vi "Lab Panel V5.24.1.vi"() -> ()   [LabVIEW 2013] (continued)
                n1784 = property on="O/I  LAB02-2" class="Bool (strict)"("DisabledEnum"=w3327) -> ()  [unwired: 2 in, 2 out]
                n1785 = property on="O/I  LAB03-1" class="Bool (strict)"("DisabledEnum"=w3326) -> ()  [unwired: 2 in, 2 out]
              }
              frame #1 {
                n1786 = Select(t=2, s=w3360, f=0) -> (s? t:f=w3351:i32)
                n1787 = Select(t=2, s=w3359, f=0) -> (s? t:f=w3352:i32)
                n1788 = Select(t=2, s=w3356, f=0) -> (s? t:f=w3355:i32)
                n1789 = Select(t=2, s=w3357, f=0) -> (s? t:f=w3354:i32)
                n1790 = Select(t=2, s=w3358, f=0) -> (s? t:f=w3353:i32)
                n1791 = property on="SELECT LAB05-2" class="RadioBtnsControl (strict)"("DisabledEnum"=w3351) -> ()  [unwired: 2 in, 2 out]
                n1792 = property on="SELECT LAB05-1" class="RadioBtnsControl (strict)"("DisabledEnum"=w3352) -> ()  [unwired: 2 in, 2 out]
                n1793 = property on="SELECT LAB03-2" class="RadioBtnsControl (strict)"("DisabledEnum"=w3355) -> ()  [unwired: 2 in, 2 out]
                n1794 = property on="SELECT LAB04-1" class="RadioBtnsControl (strict)"("DisabledEnum"=w3354) -> ()  [unwired: 2 in, 2 out]
                n1795 = property on="SELECT LAB04-2" class="RadioBtnsControl (strict)"("DisabledEnum"=w3353) -> ()  [unwired: 2 in, 2 out]
                n1796 = property on="SET LAB05-2" class="Clust (strict)"("DisabledEnum"=w3351) -> ()  [unwired: 2 in, 2 out]
                n1797 = property on="SET LAB05-1" class="Clust (strict)"("DisabledEnum"=w3352) -> ()  [unwired: 2 in, 2 out]
                n1798 = property on="SET LAB03-2" class="Clust (strict)"("DisabledEnum"=w3355) -> ()  [unwired: 2 in, 2 out]
                n1799 = property on="SET LAB04-1" class="Clust (strict)"("DisabledEnum"=w3354) -> ()  [unwired: 2 in, 2 out]
                n1800 = property on="SET LAB04-2" class="Clust (strict)"("DisabledEnum"=w3353) -> ()  [unwired: 2 in, 2 out]
                n1801 = property on="O/I  LAB05-2" class="Bool (strict)"("DisabledEnum"=w3351) -> ()  [unwired: 2 in, 2 out]
                n1802 = property on="O/I  LAB05-1" class="Bool (strict)"("DisabledEnum"=w3352) -> ()  [unwired: 2 in, 2 out]
                n1803 = property on="O/I  LAB04-1" class="Bool (strict)"("DisabledEnum"=w3354) -> ()  [unwired: 2 in, 2 out]
                n1804 = property on="O/I  LAB04-2" class="Bool (strict)"("DisabledEnum"=w3353) -> ()  [unwired: 2 in, 2 out]
                n1805 = property on="O/I  LAB03-2" class="Bool (strict)"("DisabledEnum"=w3355) -> ()  [unwired: 2 in, 2 out]
                n1806 = Not(x=w3360) -> (.not. x?=w3361:bool)
                n1807 = Not(x=w3359) -> (.not. x?=w3362:bool)
                n1808 = Not(x=w3358) -> (.not. x?=w3363:bool)
                n1809 = property on="RESULT LAB05-2" class="Bool (strict)"("Visible"=w3361) -> ()  [unwired: 2 in, 2 out]
                n1810 = property on="RESULT LAB05-1" class="Bool (strict)"("Visible"=w3362) -> ()  [unwired: 2 in, 2 out]
                n1811 = Not(x=w3357) -> (.not. x?=w3364:bool)
                n1812 = property on="RESULT LAB04-2" class="Bool (strict)"("Visible"=w3363) -> ()  [unwired: 2 in, 2 out]
                n1813 = Not(x=w3356) -> (.not. x?=w3365:bool)
                n1814 = property on="RESULT LAB04-1" class="Bool (strict)"("Visible"=w3364) -> ()  [unwired: 2 in, 2 out]
                n1815 = property on="RESULT LAB03-2" class="Bool (strict)"("Visible"=w3365) -> ()  [unwired: 2 in, 2 out]
              }
              frame #2 {
                # "disable calibrate if any test running"
                n1816 = Or(x=w3388, y=w3387) -> (x .or. y?=w3381:bool)
                n1817 = Or(x=w3390, y=w3389) -> (x .or. y?=w3383:bool)
                n1818 = Or(x=w3394, y=w3393) -> (x .or. y?=w3385:bool)
                n1819 = Or(x=w3392, y=w3391) -> (x .or. y?=w3384:bool)
                n1820 = Or(x=w3396, y=w3395) -> (x .or. y?=w3386:bool)
                n1821 = Or(x=w3384, y=w3383) -> (x .or. y?=w3382:bool)
                n1822 = Or(x=w3386, y=w3385) -> (x .or. y?=w3380:bool)
                n1823 = Or(x=w3382, y=w3381) -> (x .or. y?=w3379:bool)
                n1824 = Or(x=w3380, y=w3379) -> (x .or. y?=w3376:bool)
                "Any Test Running" <- w3376
                n1825 = case shown="False" w3376 {
                  tunnel: [0 2] -> w3378
                  frame False {
                  }
                  frame True {
                  }
                }
                n1826 = property on="JIG TEST" class="Clust (strict)"("DisabledEnum"=w3378) -> ()  [unwired: 2 in, 2 out]
                n1827 = property on="Network Directory" class="Path"("DisabledEnum"=w3378) -> ()  [unwired: 2 in, 2 out]
                n1828 = property on="MAIL SETTINGS" class="Clust (strict)"("DisabledEnum"=w3378) -> ()  [unwired: 2 in, 2 out]
                n1829 = property on="SET (cal)" class="Bool (strict)"("DisabledEnum"=w3378) -> ()  [unwired: 2 in, 2 out]
                n1830 = property on="ADMIN" class="Bool (strict)"("DisabledEnum"=0) -> ()  [unwired: 2 in, 2 out]
              }
            }
          }
          frame #8 {
            # "drive jigs"
            n1831 = stacked-sequence {
              frame #0 {
                # "jig on"
                n1832 = local read "jig cycle"() -> (w3404:dbl)
                n1833 = property on="JIG TEST" class="Clust (strict)"() -> ("DisabledEnum"=w3401:T16)  [unwired: 2 in, 2 out]
                n1834 = Equal?(x=w3401, y=2) -> (x = y?=w3400:bool)
                n1835 = Equal?(x=w3404, y=0) -> (x = y?=w3402:bool)
                n1836 = And(x=w3402, y=w3400) -> (x .and. y?=w3399:bool)
                n1837 = case shown="True" w3399 {
                  frame False {
                  }
                  frame True {
                    n1838 = local read "run lab01-1"() -> (w3415:bool)
                    n1839 = local read "run lab01-2"() -> (w3414:bool)
                    n1840 = local read "run lab02-1"() -> (w3413:bool)
                    n1841 = local read "run lab02-2"() -> (w3412:bool)
                    n1842 = local read "run lab03-1"() -> (w3411:bool)
                    n1843 = local read "run lab03-2"() -> (w3410:bool)
                    n1844 = local read "run lab04-1"() -> (w3409:bool)
                    n1845 = local read "run lab04-2"() -> (w3408:bool)
                    n1846 = local read "run lab05-1"() -> (w3407:bool)
                    n1847 = local read "run lab05-2"() -> (w3406:bool)
                    n1848 = local write "JIG LAB03-2"(w3410) -> ()
                    n1849 = local write "JIG LAB01-1"(w3415) -> ()
                    n1850 = local write "JIG LAB01-2"(w3414) -> ()
                    n1851 = local write "JIG LAB02-1"(w3413) -> ()
                    n1852 = local write "JIG LAB02-2"(w3412) -> ()
                    n1853 = local write "JIG LAB03-1"(w3411) -> ()
                    n1854 = local write "JIG LAB04-1"(w3409) -> ()
                    n1855 = local write "JIG LAB04-2"(w3408) -> ()
                    n1856 = local write "JIG LAB05-1"(w3407) -> ()
                    n1857 = local write "JIG LAB05-2"(w3406) -> ()
                  }
                }
              }
              frame #1 {
                # "jig off"
                n1858 = local read "jig cycle"() -> (w3422:dbl)
                n1859 = local read "on loops"() -> (w3421:dbl)
                n1860 = property on="JIG TEST" class="Clust (strict)"() -> ("DisabledEnum"=w3420:T16)  [unwired: 2 in, 2 out]
                n1861 = Equal?(x=w3420, y=2) -> (x = y?=w3418:bool)
                n1862 = Equal?(x=w3422, y=w3421) -> (x = y?=w3417:bool)
                n1863 = And(x=w3417, y=w3418) -> (x .and. y?=w3416:bool)
                n1864 = case shown="True" w3416 {
                  frame False {
                  }
                  frame True {
                    w3473 = FALSE
                    w3474 = TRUE
                    w3472 = 2
                    n1865 = local read "SELECT LAB05-2"() -> (w3463:T3)
                    n1866 = local read "SELECT LAB04-2"() -> (w3465:T3)
                    n1867 = local read "SELECT LAB04-1"() -> (w3466:T3)
                    n1868 = local read "SELECT LAB05-1"() -> (w3464:T3)
                    n1869 = local read "SELECT LAB03-2"() -> (w3467:T3)
                    n1870 = local read "SELECT LAB02-1"() -> (w3470:T3)
                    n1871 = local read "SELECT LAB03-1"() -> (w3468:T3)
                    n1872 = local read "SELECT LAB02-2"() -> (w3469:T3)
                    n1873 = local read "SELECT LAB01-2"() -> (w3471:T3)
                    n1874 = local read "run lab05-1"() -> (w3433:bool)
                    n1875 = local read "run lab05-2"() -> (w3432:bool)
                    n1876 = local read "SELECT LAB01-1"() -> (w3475:T3)
                    n1877 = local read "run lab04-2"() -> (w3434:bool)
                    n1878 = local read "run lab04-1"() -> (w3435:bool)
                    n1879 = local read "run lab01-1"() -> (w3451:bool)
                    n1880 = local read "run lab01-2"() -> (w3440:bool)
                    n1881 = local read "run lab03-2"() -> (w3436:bool)
                    n1882 = local read "run lab03-1"() -> (w3437:bool)
                    n1883 = local read "run lab02-1"() -> (w3439:bool)
                    n1884 = local read "run lab02-2"() -> (w3438:bool)
                    n1885 = Equal?(x=w3472, y=w3468) -> (x = y?=w3446:bool)
                    n1886 = Equal?(x=w3472, y=w3467) -> (x = y?=w3445:bool)
                    n1887 = Equal?(x=w3472, y=w3466) -> (x = y?=w3444:bool)
                    n1888 = Equal?(x=w3472, y=w3465) -> (x = y?=w3443:bool)
                    n1889 = Equal?(x=w3472, y=w3464) -> (x = y?=w3442:bool)
                    n1890 = Equal?(x=w3472, y=w3463) -> (x = y?=w3441:bool)
                    n1891 = Equal?(x=w3472, y=w3475) -> (x = y?=w3452:bool)
                    n1892 = Equal?(x=w3472, y=w3470) -> (x = y?=w3448:bool)
                    n1893 = Equal?(x=w3472, y=w3469) -> (x = y?=w3447:bool)
                    n1894 = Equal?(x=w3472, y=w3471) -> (x = y?=w3449:bool)
                    n1895 = And(x=w3443, y=w3434) -> (x .and. y?=w3425:bool)
                    n1896 = And(x=w3446, y=w3437) -> (x .and. y?=w3428:bool)
                    n1897 = And(x=w3444, y=w3435) -> (x .and. y?=w3426:bool)
                    n1898 = And(x=w3441, y=w3432) -> (x .and. y?=w3423:bool)
                    n1899 = And(x=w3447, y=w3438) -> (x .and. y?=w3429:bool)
                    n1900 = And(x=w3445, y=w3436) -> (x .and. y?=w3427:bool)
                    n1901 = And(x=w3442, y=w3433) -> (x .and. y?=w3424:bool)
                    n1902 = And(x=w3449, y=w3440) -> (x .and. y?=w3431:bool)
                    n1903 = And(x=w3452, y=w3451) -> (x .and. y?=w3450:bool)
                    n1904 = And(x=w3448, y=w3439) -> (x .and. y?=w3430:bool)
                    n1905 = Select(t=w3474, s=w3450, f=w3473) -> (s? t:f=w3453:bool)
                    n1906 = Select(t=w3474, s=w3431, f=w3473) -> (s? t:f=w3454:bool)
                    n1907 = Select(t=w3474, s=w3430, f=w3473) -> (s? t:f=w3455:bool)
                    n1908 = Select(t=w3474, s=w3429, f=w3473) -> (s? t:f=w3456:bool)
                    n1909 = Select(t=w3474, s=w3428, f=w3473) -> (s? t:f=w3457:bool)
                    n1910 = Select(t=w3474, s=w3427, f=w3473) -> (s? t:f=w3458:bool)
                    n1911 = Select(t=w3474, s=w3426, f=w3473) -> (s? t:f=w3459:bool)
                    n1912 = Select(t=w3474, s=w3425, f=w3473) -> (s? t:f=w3460:bool)
                    n1913 = Select(t=w3474, s=w3424, f=w3473) -> (s? t:f=w3461:bool)
                    n1914 = Select(t=w3474, s=w3423, f=w3473) -> (s? t:f=w3462:bool)
                    n1915 = local write "JIG LAB03-2"(w3458) -> ()
                    n1916 = local write "JIG LAB02-1"(w3455) -> ()
                    n1917 = local write "JIG LAB02-2"(w3456) -> ()
                    n1918 = local write "JIG LAB01-2"(w3454) -> ()
                    n1919 = local write "JIG LAB03-1"(w3457) -> ()
                    n1920 = local write "JIG LAB01-1"(w3453) -> ()
                    n1921 = local write "JIG LAB05-2"(w3462) -> ()
                    n1922 = local write "JIG LAB04-1"(w3459) -> ()
                    n1923 = local write "JIG LAB05-1"(w3461) -> ()
                    n1924 = local write "JIG LAB04-2"(w3460) -> ()
                  }
                }
              }
            }
          }
          frame #9 {
            # "enable  jig test output if no test busy"
            n1925 = property on="JIG TEST" class="Clust (strict)"() -> ("DisabledEnum"=w3478:T16)  [unwired: 2 in, 2 out]
            n1926 = Equal?(x=w3478, y=0) -> (x = y?=w3476:bool)
            n1927 = case shown="True" w3476 {
              frame False {
              }
              frame True {
                n1928 = local read "JIG TEST"() -> (w3489:T10)
                n1929 = Unbundle(w3489) -> ("LAB01-1"=w3488:bool, "LAB01-2"=w3487:bool, "LAB02-1"=w3486:bool, "LAB02-2"=w3485:bool, "LAB03-1"=w3484:bool, "LAB03-2"=w3483:bool, "LAB04-1"=w3482:bool, "LAB04-2"=w3481:bool, "LAB05-1"=w3480:bool, "LAB05-2"=w3479:bool)
                n1930 = local write "JIG LAB05-1"(w3480) -> ()
                n1931 = local write "JIG LAB05-2"(w3479) -> ()
                n1932 = local write "JIG LAB04-1"(w3482) -> ()
                n1933 = local write "JIG LAB04-2"(w3481) -> ()
                n1934 = local write "JIG LAB03-2"(w3483) -> ()
                n1935 = local write "JIG LAB01-1"(w3488) -> ()
                n1936 = local write "JIG LAB02-1"(w3486) -> ()
                n1937 = local write "JIG LAB03-1"(w3484) -> ()
                n1938 = local write "JIG LAB01-2"(w3487) -> ()
                n1939 = local write "JIG LAB02-2"(w3485) -> ()
              }
            }
          }
          frame #10 {
            w3490 = FALSE
            # "Drive digital output and reset USB and temperature network if required."
            n1940 = global read "Global display 3.vi" "cycle O/F"() -> (w3499:bool)
            n1941 = local read "O/I  LAB05-2"() -> (w3492:bool)
            n1942 = local read "O/I  LAB05-1"() -> (w3494:bool)
            n1943 = local read "JIG LAB05-2"() -> (w3491:bool)
            n1944 = local read "O/I  LAB04-2"() -> (w3496:bool)
            n1945 = local read "JIG LAB05-1"() -> (w3493:bool)
            n1946 = local read "JIG LAB04-2"() -> (w3495:bool)
            n1947 = local read "O/I  LAB03-1"() -> (w3510:bool)
            n1948 = local read "O/I  LAB04-1"() -> (w3506:bool)
            n1949 = local read "O/I  LAB02-1"() -> (w3514:bool)
            n1950 = local read "O/I  LAB02-2"() -> (w3512:bool)
            n1951 = local read "O/I  LAB03-2"() -> (w3508:bool)
            n1952 = local read "JIG LAB04-1"() -> (w3505:bool)
            n1953 = local read "JIG LAB03-2"() -> (w3507:bool)
            n1954 = local read "O/I  LAB01-2"() -> (w3516:bool)
            n1955 = local read "JIG LAB02-1"() -> (w3513:bool)
            n1956 = local read "JIG LAB02-2"() -> (w3511:bool)
            n1957 = local read "JIG LAB03-1"() -> (w3509:bool)
            n1958 = local read "O/I  LAB01-1"() -> (w3518:bool)
            n1959 = local read "JIG LAB01-2"() -> (w3515:bool)
            n1960 = local read "JIG LAB01-1"() -> (w3517:bool)
            n1961 = case shown="False" w3499 {
              tunnel: [w3622 FALSE] -> w3498
              frame False {
                n1962 = local read "Analog error"() -> (w3624:bool)
                n1963 = local read "Reset Measuring"() -> (w3623:bool)
                n1964 = Or(x=w3623, y=w3624) -> (x .or. y?=w3622:bool)
              }
              frame True {
              }
            }
            n1965 = Build Array(w3511, w3510, w3509, w3508, w3507, w3506, w3505) -> (w3503:bool[])
            "USB OUT 1" <- w3503
            n1966 = Build Array(w3518, w3517, w3516, w3515, w3514, w3513, w3512) -> (w3504:bool[])
            "USB OUT 0" <- w3504
            n1967 = Build Array(w3496, w3495, w3494, w3493, w3492, w3491, w3490, w3490) -> (w3502:bool[])
            "USB OUT 2" <- w3502
            n1968 = Not(x=w3499) -> (.not. x?=w3500:bool)
            n1969 = local read "Simulate"() -> (w3501:bool)
            n1970 = And(x=w3500, y=w3498) -> (x .and. y?=w3497:bool)
            n1971 = stacked-sequence {
              tunnel: w3504 -> [w3522 w3528]
              tunnel: w3503 -> [w3521 w3527]
              tunnel: w3502 -> [w3520 w3526]
              tunnel: w3501 -> [w3519 w3529]
              tunnel: w3497 -> [_ w3530]
              frame #0 {
                # "drive outputs for normal use"
                n1972 = case shown="False" w3519 {
                  tunnel: w3522 -> [w3525 _]
                  tunnel: w3521 -> [w3524 _]
                  tunnel: w3520 -> [w3523 _]
                  frame False {
                    n1973 = call "sub vi - Drive Relays All v6.vi"("Array #2"=w3523, "Array #1"=w3524, "Array #0"=w3525) -> ()  [unwired: 8 in, 1 out]
                  }
                  frame True {
                  }
                }
              }
              frame #1 {
                # "USB  reset routine"
                n1974 = case shown="True" w3530 {
                  tunnel: w3529 -> [_ w3534]
                  tunnel: w3528 -> [_ w3533]
                  tunnel: w3527 -> [_ w3532]
                  tunnel: w3526 -> [_ w3531]
                  frame False {
                  }
                  frame True {
                    n1975 = stacked-sequence {
                      seq-local: [w3536 _ _ _ _] -> [_ w3542 _ _ _]
                      tunnel: w3534 -> [_ w3546 _ _ _]
                      tunnel: w3533 -> [_ w3545 _ _ _]
                      tunnel: w3532 -> [_ w3544 _ _ _]
                      tunnel: w3531 -> [_ w3543 _ _ _]
                      frame #0 {
                        n1976 = case shown="False" "Auto Reset" {
                          tunnel: [w3539 FALSE] -> w3537
                          frame False {
                            n1977 = Two Button Dialog(message="System reset") -> (T button?=w3539:bool)  [unwired: 2 in]
                          }
                          frame True {
                          }
                        }
                        n1978 = disable-structure shown="Disabled" {
                          frame Disabled {
                            n1979 = local write "Tab Control 2"(5) -> ()
                          }
                          frame Enabled {
                          }
                        }
                        n1980 = Or(x="Auto Reset", y=w3537) -> (x .or. y?=w3536:bool)
                      }
                      frame #1 {
                        n1981 = case shown="True" w3542 {
                          tunnel: w3546 -> [_ w3552]
                          tunnel: w3545 -> [_ w3551]
                          tunnel: w3544 -> [_ w3550]
                          tunnel: w3543 -> [_ w3549]
                          frame False {
                          }
                          frame True {
                            n1982 = stacked-sequence {
                              tunnel: w3552 -> [_ w3570 _]
                              tunnel: bool[] [] -> [w3555 w3569 w3579]
                              tunnel: w3551 -> [_ _ w3578]
                              tunnel: w3550 -> [w3554 _ w3577]
                              tunnel: w3549 -> [w3553 _ w3576]
                              tunnel: 5000 -> [w3556 _ w3575]
                              frame #0 {
                                # "switch off test stations for system reset"
                                n1983 = stacked-sequence {
                                tunnel: w3556 -> [w3560 w3564 w3566]
                                tunnel: w3555 -> [w3559 w3563 w3567]
                                tunnel: w3554 -> [w3558 _ _]
                                tunnel: w3553 -> [w3557 w3562 _]
                                frame #0 {
                                # "drive 1st 7 inputs"
                                n1984 = call "sub vi - Drive Relays All v6.vi"("Array #2"=w3557, "Array #1"=w3558, "Array #0"=w3559) -> ()  [unwired: 8 in, 1 out]
                                n1985 = call "Message Display V1.vi"("Message"="Delay off LAB 01-1 to 02-1", "Delay mS"=w3560) -> ()  [unwired: 10 in]
                                }
                                frame #1 {
                                # "drive 2nd 7 inputs"
                                n1986 = call "sub vi - Drive Relays All v6.vi"("Array #2"=w3562, "Array #1"=w3563, "Array #0"=w3563) -> ()  [unwired: 8 in, 1 out]
                                n1987 = call "Message Display V1.vi"("Message"="Delay off LAB 02-2 to 04-1", "Delay mS"=w3564) -> ()  [unwired: 10 in]
                                }
                                frame #2 {
                                # "drive 3rd 7 inputs"
                                n1988 = call "sub vi - Drive Relays All v6.vi"("Array #2"=w3567, "Array #1"=w3567, "Array #0"=w3567) -> ()  [unwired: 8 in, 1 out]
                                n1989 = call "Message Display V1.vi"("Message"="Delay off LAB 04-2 to 05-2", "Delay mS"=w3566) -> ()  [unwired: 10 in]
                                }
                                }
                              }
                              frame #1 {
                                # "reset all usb modules"
                                n1990 = stacked-sequence {
                                tunnel: w3570 -> [_ w3574]
                                tunnel: w3569 -> [w3572 _]
                                frame #0 {
                                n1991 = call "sub vi - Drive Relays All v6.vi"("Array #2"=bool[] [FALSE, FALSE, FALSE, FALSE, FALSE, FALSE, TRUE, FALSE], "Array #1"=w3572, "Array #0"=w3572) -> ()  [unwired: 8 in, 1 out]
                                }
                                frame #1 {
                                n1992 = call "Reset Meas v 4.vi"("simulate"=w3574) -> ("Reset Error"=→"Reset Error":bool)  [unwired: 10 in]
                                }
                                }
                              }
                              frame #2 {
                                # "switch test stations back on after reset"
                                n1993 = stacked-sequence {
                                tunnel: w3579 -> [w3583 w3586 _]
                                tunnel: w3578 -> [w3582 w3588 w3593]
                                tunnel: w3575 -> [w3581 w3584 w3590]
                                tunnel: w3577 -> [_ w3587 w3592]
                                tunnel: w3576 -> [_ _ w3589]
                                frame #0 {
                                # "drive 1st 7 inputs"
                                n1994 = call "sub vi - Drive Relays All v6.vi"("Array #2"=w3583, "Array #1"=w3583, "Array #0"=w3582) -> ()  [unwired: 8 in, 1 out]
                                n1995 = call "Message Display V1.vi"("Message"="Delay on LAB 01-1 to 02-1", "Delay mS"=w3581) -> ()  [unwired: 10 in]
                                }
                                frame #1 {
                                # "drive 1st & 2nd outputs"
                                n1996 = call "sub vi - Drive Relays All v6.vi"("Array #2"=w3586, "Array #1"=w3587, "Array #0"=w3588) -> ()  [unwired: 8 in, 1 out]
                                n1997 = call "Message Display V1.vi"("Message"="Delay on LAB 02-2 to 04-1", "Delay mS"=w3584) -> ()  [unwired: 10 in]
                                }
                                frame #2 {
                                n1998 = call "sub vi - Drive Relays All v6.vi"("Array #2"=w3589, "Array #1"=w3592, "Array #0"=w3593) -> ()  [unwired: 8 in, 1 out]
                                n1999 = call "Message Display V1.vi"("Message"="Delay on LAB 04-2 to 05-2", "Delay mS"=w3590) -> ()  [unwired: 10 in]
                                }
                                }
                              }
                            }
                          }
                        }
                      }
                      frame #2 {
                        w3594 = 0
                        w3595 = FALSE
                        # "set all back to zero"
                        n2000 = local read "Total USB resets"() -> (w3597:dbl)
                        n2001 = local read "Resets Done"() -> (w3599:dbl)
                        n2002 = local write "Reset Measuring"(w3595) -> ()
                        n2003 = local write "Analog error"(w3595) -> ()
                        n2004 = local write "Er USB#2"(w3594) -> ()
                        n2005 = local write "Er USB#0"(w3594) -> ()
                        n2006 = local write "Er USB#1"(w3594) -> ()
                        n2007 = local write "Error USB #0"(w3595) -> ()
                        n2008 = local write "Error USB #1"(w3595) -> ()
                        n2009 = local write "Error USB #2"(w3595) -> ()
                        n2010 = Increment(x=w3597) -> (x+1=w3596:dbl)
                        n2011 = Increment(x=w3599) -> (x+1=→"Resets Done":dbl)
                        n2012 = local write "Total USB resets"(w3596) -> ()
                      }
                      frame #3 {
                        # "save reset value"
                        n2013 = String To Path(string="c:\\crabtree\\Set Up\\") -> (path=w3609:path)
                        n2014 = Build Path(base path=w3609, name or relative path="USB resets.bin") -> (appended path=w3602:path)
                        n2015 = Create Folder(path (use dialog)=w3609) -> (error out=w3601:errorcluster)  [unwired: 2 in, 2 out]
                        n2016 = local read "Total USB resets"() -> (w3600:dbl)
                        n2017 = call <vilib>:"Clear Errors.vi"("error in (no error)"=w3601) -> ()  [unwired: 6 in, 1 out]
                        n2018 = Open/Create/Replace File(file path (use dialog)=w3602, operation (0:open)=T17."replace or create") -> (refnum out=w3607:refnum<file>, error out=w3606:errorcluster)  [unwired: 4 in, 1 out]
                        n2019 = Write to Binary File(file (use dialog)=w3607, data=w3600, error in=w3606) -> (refnum out=w3605:refnum<file>, error out=w3604:errorcluster)  [unwired: 3 in, 1 out]
                        n2020 = Close File(refnum=w3605, error in=w3604) -> (error out=w3603:errorcluster)  [unwired: 1 out]
                        n2021 = local write "data file error"(w3603) -> ()
                      }
                      frame #4 {
                        # "mail reset value"
                        n2022 = local read "Total USB resets"() -> (w3618:dbl)
                        n2023 = local read "MAIL SETTINGS"() -> (w3614:T7)
                        n2024 = local read "Mail Test File To:"() -> (w3619:string)
                        n2025 = Number To Decimal String(number=w3618) -> (decimal integer string=w3616:string)  [unwired: 1 in]
                        n2026 = Unbundle(w3614) -> ("OUT SERVER ADDRESS"=w3621:string, "FROM ACCOUNT"=w3620:string)  [unwired: 5 out]
                        n2027 = Concatenate Strings("Total USB resets: ", w3616) -> (w3615:string)
                        n2028 = call "sub vi - send mail v5.vi"("TO:"=w3619, "subject"=w3615, "from"=w3620, "out going server"=w3621) -> ("error out"=w3613:errorcluster)  [unwired: 11 in]
                        n2029 = Bundle(cluster=w3614, "mail error"=w3613) -> (w3612:T7)  [unwired: 6 in]
                        n2030 = local write "MAIL SETTINGS"(w3612) -> ()
                      }
                    }
                  }
                }
              }
            }
          }
          frame #11 {
            # "if all test panels are off stop analog read"
            n2031 = local read "O/I  LAB03-1"() -> (w3642:bool)
            n2032 = local read "O/I  LAB03-2"() -> (w3641:bool)
            n2033 = local read "O/I  LAB04-1"() -> (w3640:bool)
            n2034 = local read "O/I  LAB04-2"() -> (w3639:bool)
            n2035 = local read "O/I  LAB05-1"() -> (w3638:bool)
            n2036 = local read "O/I  LAB05-2"() -> (w3637:bool)
            n2037 = local read "O/I  LAB02-2"() -> (w3643:bool)
            n2038 = local read "O/I  LAB02-1"() -> (w3644:bool)
            n2039 = local read "O/I  LAB01-2"() -> (w3645:bool)
            n2040 = local read "O/I  LAB01-1"() -> (w3646:bool)
            n2041 = Or(x=w3638, y=w3637) -> (x .or. y?=w3635:bool)
            n2042 = Or(x=w3640, y=w3639) -> (x .or. y?=w3636:bool)
            n2043 = Or(x=w3644, y=w3643) -> (x .or. y?=w3634:bool)
            n2044 = Or(x=w3642, y=w3641) -> (x .or. y?=w3632:bool)
            n2045 = Or(x=w3646, y=w3645) -> (x .or. y?=w3633:bool)
            n2046 = Or(x=w3636, y=w3635) -> (x .or. y?=w3629:bool)
            n2047 = Or(x=w3633, y=w3634) -> (x .or. y?=w3631:bool)
            n2048 = Or(x=w3631, y=w3632) -> (x .or. y?=w3630:bool)
            n2049 = local read "Any Test Running"() -> (w3628:bool)
            n2050 = Or(x=w3630, y=w3629) -> (x .or. y?=w3627:bool)
            n2051 = Or(x=w3627, y=w3628) -> (x .or. y?=w3626:bool)
          }
          frame #12 {
            # "get all analog values from USB devices"
            n2052 = local read "on loops"() -> (w3654:dbl)
            n2053 = local read "jig cycle"() -> (w3651:dbl)
            n2054 = Add(x=w3654, y=1) -> (x+y=w3652:dbl)
            n2055 = Equal?(x=w3651, y=1) -> (x = y?=w3649:bool)
            n2056 = Equal?(x=w3651, y=w3652) -> (x = y?=w3650:bool)
            n2057 = Or(x=w3649, y=w3650) -> (x .or. y?=w3648:bool)
            n2058 = global write "Global display 3.vi" "cycle O/F"(w3649) -> ()
            n2059 = case shown="True" w3648 {
              tunnel: w3649 -> [_ w3659]
              tunnel: w3647 -> [_ w3656]
              frame False {
              }
              frame True {
                n2060 = local read "Simulate"() -> (w3662:bool)
                n2061 = case shown="False" w3662 {
                  tunnel: [w3679 0.3 ("Analog loop time")] -> w3669
                  tunnel: [w3678 dynamicdata[] [] ("array GRAPH")] -> w3668
                  tunnel: [w3677 w3699] -> w3667
                  tunnel: [w3676 w3699] -> w3666
                  tunnel: [w3675 w3699] -> w3665
                  tunnel: [w3674 w3699] -> w3664
                  tunnel: [w3673 w3699] -> w3663
                  tunnel: w3659 -> [_ w3703]
                  tunnel: [w3672 "Ambient Volts"] -> w3658
                  tunnel: [w3671 bool[] []] -> w3657
                  tunnel: w3656 -> [w3670 _]
                  frame False {
                    # "analog in"
                    n2062 = case shown="True" w3670 {
                      tunnel: [0 w3694] -> w3679
                      tunnel: [dynamicdata[] [] ("array GRAPH") w3693] -> w3678
                      tunnel: [w3680 w3692] -> w3677
                      tunnel: [w3680 w3691] -> w3676
                      tunnel: [w3680 w3690] -> w3675
                      tunnel: [w3680 w3689] -> w3674
                      tunnel: [w3680 w3688] -> w3673
                      tunnel: [3 w3687] -> w3672
                      tunnel: [bool[] [] w3686] -> w3671
                      frame False {
                        w3681 = 0.0
                        # "no test"
                        n2063 = Bundle(w3681, w3681, w3681, w3681, w3681, w3681) -> (w3680:cluster{dbl, dbl, dbl, dbl, dbl, dbl})  [unwired: 1 in]
                      }
                      frame True {
                        # "test on"
                        n2064 = call "sub vi - Read Analog All v9.3.vi"() -> ("Analog loop time"=w3694:dbl, "array GRAPH"=w3693:dynamicdata[], "LAB01"=w3692:T27, "LAB02"=w3691:T28, "LAB03"=w3690:T29, "LAB04"=w3689:T30, "deg C"=w3687:dbl, "USB Error"=w3686:bool[], "LAB05"=w3688:T31)  [unwired: 7 in]
                      }
                    }
                  }
                  frame True {
                    # "simulate"
                    n2065 = local read "ON amps"() -> (w3697:dbl)
                    n2066 = local read "OFF amps"() -> (w3698:dbl)
                    n2067 = local read "VOLTS"() -> (w3701:dbl)
                    n2068 = local read "PF"() -> (w3700:dbl)
                    n2069 = Select(t=w3697, s=w3703, f=w3698) -> (s? t:f=w3702:dbl)
                    n2070 = Bundle("OFF amps"=w3702, "VOLTS"=w3701, "PF"=w3700, "OFF amps"=w3702, "VOLTS"=w3701, "PF"=w3700) -> (w3699:T32)  [unwired: 1 in]
                  }
                }
                n2071 = local read "Simulate"() -> (w3661:bool)
                n2072 = stacked-sequence {
                  seq-local: [w3708 _ _ _ _ _ _ _] -> [_ _ _ _ _ _ _ _]
                  seq-local: [w3707 _ _ _ _ _ _ _] -> [_ _ _ _ _ _ _ _]
                  seq-local: [w3706 _ _ _ _ _ _ _] -> [_ _ _ _ _ _ _ w3903]
                  tunnel: w3669 -> [_ w3761 _ _ _ _ _ _]
                  tunnel: w3668 -> [_ w3758 _ _ _ _ _ _]
                  tunnel: w3667 -> [_ _ w3788 _ _ _ _ _]
                  tunnel: w3666 -> [_ _ _ w3816 _ _ _ _]
                  tunnel: w3665 -> [_ _ _ _ w3844 _ _ _]
                  tunnel: w3664 -> [_ _ _ _ _ w3872 _ _]
                  tunnel: w3663 -> [_ _ _ _ _ _ w3900 _]
                  tunnel: w3661 -> [_ _ w3787 w3815 w3843 w3871 w3899 w3905]
                  tunnel: T14 {"1  (A) cal"=1.0, "1 (V) cal"=1.0, "1 (PF) cal"=1.0, "1 (TL) cal"=1.0, "1 (TN) cal"=1.0, "2 (A) cal"=1.0, "2 (V) cal"=1.0, "2 (PF) cal"=1.0, "2 (TL) cal"=1.0, "2 (TN) cal"=1.0} ("CAL LAB01") -> [_ _ w3786 w3814 w3842 w3870 w3898 _]
                  tunnel: w3658 -> [_ _ _ _ _ _ _ w3904]
                  tunnel: w3657 -> [w3711 _ _ _ _ _ _ _]
                  frame #0 {
                    n2073 = Index Array(array=w3711, index=2) -> (element=w3706:bool)
                    n2074 = Index Array(array=w3711, index=1) -> (element=w3707:bool)
                    n2075 = Index Array(array=w3711, index=0) -> (element=w3708:bool)
                    n2076 = local write "Error USB #2"(w3706) -> ()
                    n2077 = local write "Error USB #0"(w3708) -> ()
                    n2078 = local write "Error USB #1"(w3707) -> ()
                    n2079 = stacked-sequence {
                      tunnel: w3708 -> [w3715 _ _ _]
                      tunnel: w3707 -> [_ w3720 _ _]
                      tunnel: 0 -> [w3714 w3719 w3724 _]
                      tunnel: w3706 -> [_ _ w3725 _]
                      frame #0 {
                        n2080 = case shown="True" w3715 {
                          tunnel: w3714 -> [w3716 _]
                          frame False {
                            n2081 = local write "Er USB#0"(w3716) -> ()
                          }
                          frame True {
                            n2082 = local read "Er USB#0"() -> (w3718:dbl)
                            n2083 = Increment(x=w3718) -> (x+1=→"Er USB#0":dbl)
                          }
                        }
                      }
                      frame #1 {
                        n2084 = case shown="True" w3720 {
                          tunnel: w3719 -> [w3721 _]
                          frame False {
                            n2085 = local write "Er USB#1"(w3721) -> ()
                          }
                          frame True {
                            n2086 = local read "Er USB#1"() -> (w3723:dbl)
                            n2087 = Increment(x=w3723) -> (x+1=→"Er USB#1":dbl)
                          }
                        }
                      }
                      frame #2 {
                        n2088 = case shown="True" w3725 {
                          tunnel: w3724 -> [w3726 _]
                          frame False {
                            n2089 = local write "Er USB#2"(w3726) -> ()
                          }
                          frame True {
                            n2090 = local read "Er USB#2"() -> (w3728:dbl)
                            n2091 = Increment(x=w3728) -> (x+1=→"Er USB#2":dbl)
                          }
                        }
                      }
                      frame #3 {
                        w3734 = 5
                        n2092 = local read "Er USB#2"() -> (w3735:dbl)
                        n2093 = local read "Er USB#0"() -> (w3737:dbl)
                        n2094 = local read "Er USB#1"() -> (w3736:dbl)
                        n2095 = Greater Or Equal?(x=w3737, y=w3734) -> (x >= y?=w3732:bool)
                        n2096 = Greater Or Equal?(x=w3736, y=w3734) -> (x >= y?=w3731:bool)
                        n2097 = Greater Or Equal?(x=w3735, y=w3734) -> (x >= y?=w3730:bool)
                        n2098 = Or(x=w3732, y=w3731) -> (x .or. y?=w3733:bool)
                        n2099 = Or(x=w3733, y=w3730) -> (x .or. y?=→"Analog error":bool)
                      }
                    }
                  }
                  frame #1 {
                    # "display graph data on ADM page"
                    n2100 = local write "AI"(TRUE) -> ()
                    n2101 = global write "Global 1.vi" "RATE(Hz)"("RATE (Hz)") -> ()
                    n2102 = global write "Global 1.vi" "SAMPLES"("SAMPLES") -> ()
                    n2103 = Index Array(array=w3758, index=6) -> (element=→"LAB04-1 (GRAPH)":dynamicdata)
                    n2104 = Index Array(array=w3758, index=7) -> (element=→"LAB04-2 (GRAPH)":dynamicdata)
                    n2105 = Index Array(array=w3758, index=9) -> (element=→"LAB05-2 (GRAPH)":dynamicdata)
                    n2106 = Index Array(array=w3758, index=8) -> (element=→"LAB05-1 (GRAPH)":dynamicdata)
                    n2107 = Index Array(array=w3758, index=5) -> (element=→"LAB03-2 (GRAPH)":dynamicdata)
                    n2108 = Index Array(array=w3758, index=0) -> (element=→"LAB01-1 (GRAPH)":dynamicdata)
                    n2109 = Index Array(array=w3758, index=1) -> (element=→"LAB01-2 (GRAPH)":dynamicdata)
                    n2110 = Index Array(array=w3758, index=2) -> (element=→"LAB02-1 (GRAPH)":dynamicdata)
                    n2111 = Index Array(array=w3758, index=3) -> (element=→"LAB02-2 (GRAPH)":dynamicdata)
                    n2112 = Index Array(array=w3758, index=4) -> (element=→"LAB03-1 (GRAPH)":dynamicdata)
                    "AI loop time" <- w3761
                  }
                  frame #2 {
                    n2113 = case shown="False" w3787 {
                      tunnel: [w3789 w3790] -> w3785
                      tunnel: w3786 -> [_ w3790]
                      frame False {
                        n2114 = local read "CAL LAB01"() -> (w3789:T14)
                      }
                      frame True {
                      }
                    }
                    n2115 = Unbundle By Name(w3788) -> ("OFF amps"=w3784:dbl, "VOLTS"=w3783:dbl, "PF"=w3782:dbl, "OFF amps"=w3781:dbl, "VOLTS"=w3780:dbl, "PF"=w3779:dbl)
                    n2116 = Unbundle By Name(w3785) -> ("1  (A) cal"=w3778:dbl, "1 (V) cal"=w3777:dbl, "1 (PF) cal"=w3776:dbl, "2 (A) cal"=w3775:dbl, "2 (V) cal"=w3774:dbl, "2 (PF) cal"=w3773:dbl)  [unwired: 4 out]
                    n2117 = Multiply(x=w3784, y=w3778) -> (x*y=w3771:dbl)
                    n2118 = Multiply(x=w3783, y=w3777) -> (x*y=w3770:dbl)
                    n2119 = Multiply(x=w3782, y=w3776) -> (x*y=w3769:dbl)
                    n2120 = Multiply(x=w3781, y=w3775) -> (x*y=w3767:dbl)
                    n2121 = Multiply(x=w3780, y=w3774) -> (x*y=w3766:dbl)
                    n2122 = Multiply(x=w3779, y=w3773) -> (x*y=w3765:dbl)
                    n2123 = local read "SIG LAB01-1"() -> (w3772:T2)
                    n2124 = local read "SIG LAB01-2"() -> (w3768:T2)
                    n2125 = Bundle By Name(cluster=w3772, "AMPS"=w3771, "VOLTS"=w3770, "PF"=w3769) -> (w3764:T2)
                    n2126 = Bundle By Name(cluster=w3768, "AMPS"=w3767, "VOLTS"=w3766, "PF"=w3765) -> (w3763:T2)
                    n2127 = global write "Global display 1.vi" "SIG LAB01-2"(w3763) -> ()
                    n2128 = global write "Global display 1.vi" "SIG LAB01-1"(w3764) -> ()
                    n2129 = local write "SIG LAB01-2"(w3763) -> ()
                    n2130 = local write "SIG LAB01-1"(w3764) -> ()
                  }
                  frame #3 {
                    n2131 = Unbundle By Name(w3816) -> ("OFF amps"=w3812:dbl, "VOLTS"=w3811:dbl, "PF"=w3810:dbl, "OFF amps"=w3809:dbl, "VOLTS"=w3808:dbl, "PF"=w3807:dbl)
                    n2132 = case shown="True" w3815 {
                      tunnel: [w3817 w3818] -> w3813
                      tunnel: w3814 -> [_ w3818]
                      frame False {
                        n2133 = local read "CAL LAB02"() -> (w3817:T15)
                      }
                      frame True {
                      }
                    }
                    n2134 = Unbundle By Name(w3813) -> ("1  (A) cal"=w3806:dbl, "1 (V) cal"=w3805:dbl, "1 (PF) cal"=w3804:dbl, "2 (A) cal"=w3803:dbl, "2 (V) cal"=w3802:dbl, "2 (PF) cal"=w3801:dbl)  [unwired: 4 out]
                    n2135 = Multiply(x=w3812, y=w3806) -> (x*y=w3799:dbl)
                    n2136 = Multiply(x=w3811, y=w3805) -> (x*y=w3798:dbl)
                    n2137 = Multiply(x=w3810, y=w3804) -> (x*y=w3797:dbl)
                    n2138 = Multiply(x=w3809, y=w3803) -> (x*y=w3795:dbl)
                    n2139 = Multiply(x=w3808, y=w3802) -> (x*y=w3794:dbl)
                    n2140 = Multiply(x=w3807, y=w3801) -> (x*y=w3793:dbl)
                    n2141 = local read "SIG LAB02-1"() -> (w3800:T2)
                    n2142 = local read "SIG LAB02-2"() -> (w3796:T2)
                    n2143 = Bundle By Name(cluster=w3800, "AMPS"=w3799, "VOLTS"=w3798, "PF"=w3797) -> (w3792:T2)
                    n2144 = Bundle By Name(cluster=w3796, "AMPS"=w3795, "VOLTS"=w3794, "PF"=w3793) -> (w3791:T2)
                    n2145 = global write "Global display 1.vi" "SIG LAB02-1"(w3792) -> ()
                    n2146 = local write "SIG LAB02-2"(w3791) -> ()
                    n2147 = global write "Global display 1.vi" "SIG LAB02-2"(w3791) -> ()
                    n2148 = local write "SIG LAB02-1"(w3792) -> ()
                  }
                  frame #4 {
                    n2149 = Unbundle By Name(w3844) -> ("OFF amps"=w3840:dbl, "VOLTS"=w3839:dbl, "PF"=w3838:dbl, "OFF amps"=w3837:dbl, "VOLTS"=w3836:dbl, "PF"=w3835:dbl)
                    n2150 = case shown="True" w3843 {
                      tunnel: [w3845 w3846] -> w3841
                      tunnel: w3842 -> [_ w3846]
                      frame False {
                        n2151 = local read "CAL LAB03"() -> (w3845:T14)
                      }
                      frame True {
                      }
                    }
                    n2152 = Unbundle By Name(w3841) -> ("1  (A) cal"=w3834:dbl, "1 (V) cal"=w3833:dbl, "1 (PF) cal"=w3832:dbl, "2 (A) cal"=w3831:dbl, "2 (V) cal"=w3830:dbl, "2 (PF) cal"=w3829:dbl)  [unwired: 4 out]
                    n2153 = Multiply(x=w3840, y=w3834) -> (x*y=w3827:dbl)
                    n2154 = Multiply(x=w3839, y=w3833) -> (x*y=w3821:dbl)
                    n2155 = Multiply(x=w3838, y=w3832) -> (x*y=w3826:dbl)
                    n2156 = Multiply(x=w3837, y=w3831) -> (x*y=w3824:dbl)
                    n2157 = Multiply(x=w3836, y=w3830) -> (x*y=w3823:dbl)
                    n2158 = Multiply(x=w3835, y=w3829) -> (x*y=w3822:dbl)
                    n2159 = local read "SIG LAB03-1"() -> (w3828:T2)
                    n2160 = local read "SIG LAB03-2"() -> (w3825:T2)
                    n2161 = Bundle By Name(cluster=w3828, "AMPS"=w3827, "VOLTS"=w3821, "PF"=w3826) -> (w3820:T2)
                    n2162 = Bundle By Name(cluster=w3825, "AMPS"=w3824, "VOLTS"=w3823, "PF"=w3822) -> (w3819:T2)
                    n2163 = global write "Global display 1.vi" "SIG LAB03-1"(w3820) -> ()
                    n2164 = global write "Global display 1.vi" "SIG LAB03-2"(w3819) -> ()
                    n2165 = local write "SIG LAB03-2"(w3819) -> ()
                    n2166 = local write "SIG LAB03-1"(w3820) -> ()
                  }
                  frame #5 {
                    n2167 = case shown="False" w3871 {
                      tunnel: [w3873 w3874] -> w3869
                      tunnel: w3870 -> [_ w3874]
                      frame False {
                        n2168 = local read "CAL LAB04"() -> (w3873:T14)
                      }
                      frame True {
                      }
                    }
                    n2169 = Unbundle By Name(w3872) -> ("OFF amps"=w3868:dbl, "VOLTS"=w3867:dbl, "PF"=w3866:dbl, "OFF amps"=w3865:dbl, "VOLTS"=w3864:dbl, "PF"=w3863:dbl)
                    n2170 = Unbundle By Name(w3869) -> ("1  (A) cal"=w3862:dbl, "1 (V) cal"=w3861:dbl, "1 (PF) cal"=w3860:dbl, "2 (A) cal"=w3859:dbl, "2 (V) cal"=w3858:dbl, "2 (PF) cal"=w3857:dbl)  [unwired: 4 out]
                    n2171 = Multiply(x=w3868, y=w3862) -> (x*y=w3855:dbl)
                    n2172 = Multiply(x=w3867, y=w3861) -> (x*y=w3854:dbl)
                    n2173 = Multiply(x=w3866, y=w3860) -> (x*y=w3853:dbl)
                    n2174 = Multiply(x=w3865, y=w3859) -> (x*y=w3851:dbl)
                    n2175 = Multiply(x=w3864, y=w3858) -> (x*y=w3850:dbl)
                    n2176 = Multiply(x=w3863, y=w3857) -> (x*y=w3849:dbl)
                    n2177 = local read "SIG LAB04-1"() -> (w3856:T2)
                    n2178 = local read "SIG LAB04-2"() -> (w3852:T2)
                    n2179 = Bundle By Name(cluster=w3856, "AMPS"=w3855, "VOLTS"=w3854, "PF"=w3853) -> (w3848:T2)
                    n2180 = Bundle By Name(cluster=w3852, "AMPS"=w3851, "VOLTS"=w3850, "PF"=w3849) -> (w3847:T2)
                    n2181 = global write "Global display 1.vi" "SIG LAB04-2"(w3847) -> ()
                    n2182 = global write "Global display 1.vi" "SIG LAB04-1"(w3848) -> ()
                    n2183 = local write "SIG LAB04-2"(w3847) -> ()
                    n2184 = local write "SIG LAB04-1"(w3848) -> ()
                  }
                  frame #6 {
                    n2185 = Unbundle By Name(w3900) -> ("OFF amps"=w3896:dbl, "VOLTS"=w3877:dbl, "PF"=w3895:dbl, "OFF amps"=w3894:dbl, "VOLTS"=w3893:dbl, "PF"=w3892:dbl)
                    n2186 = case shown="False" w3899 {
                      tunnel: [w3901 w3902] -> w3897
                      tunnel: w3898 -> [_ w3902]
                      frame False {
                        n2187 = local read "CAL LAB05"() -> (w3901:T14)
                      }
                      frame True {
                      }
                    }
                    n2188 = Unbundle By Name(w3897) -> ("1  (A) cal"=w3891:dbl, "1 (V) cal"=w3890:dbl, "1 (PF) cal"=w3889:dbl, "2 (A) cal"=w3888:dbl, "2 (V) cal"=w3887:dbl, "2 (PF) cal"=w3886:dbl)  [unwired: 4 out]
                    n2189 = Multiply(x=w3896, y=w3891) -> (x*y=w3884:dbl)
                    n2190 = Multiply(x=w3877, y=w3890) -> (x*y=w3883:dbl)
                    n2191 = Multiply(x=w3895, y=w3889) -> (x*y=w3882:dbl)
                    n2192 = Multiply(x=w3894, y=w3888) -> (x*y=w3880:dbl)
                    n2193 = Multiply(x=w3893, y=w3887) -> (x*y=w3879:dbl)
                    n2194 = Multiply(x=w3892, y=w3886) -> (x*y=w3878:dbl)
                    n2195 = local read "SIG LAB05-1"() -> (w3885:T2)
                    n2196 = local read "SIG LAB05-2"() -> (w3881:T2)
                    n2197 = Bundle By Name(cluster=w3885, "AMPS"=w3884, "VOLTS"=w3883, "PF"=w3882) -> (w3876:T2)
                    n2198 = Bundle By Name(cluster=w3881, "AMPS"=w3880, "VOLTS"=w3879, "PF"=w3878) -> (w3875:T2)
                    n2199 = global write "Global display 1.vi" "SIG LAB05-1"(w3876) -> ()
                    n2200 = global write "Global display 1.vi" "SIG LAB05-2"(w3875) -> ()
                    n2201 = local write "SIG LAB05-2"(w3875) -> ()
                    n2202 = local write "SIG LAB05-1"(w3876) -> ()
                  }
                  frame #7 {
                    n2203 = case shown="False" w3903 {
                      tunnel: w3905 -> [w3910 _]
                      tunnel: w3904 -> [w3909 _]
                      frame False {
                        # "update ambient referance temperature"
                        n2204 = case shown="True" w3910 {
                          tunnel: [w3912 100.0] -> w3911
                          frame False {
                            n2205 = local read "TEMP REF cal"() -> (w3912:dbl)
                          }
                          frame True {
                          }
                        }
                        n2206 = disable-structure shown="Disabled" {
                          frame Disabled {
                            n2207 = local read "Temp read loop"() -> ()  [unwired: 1 out]
                          }
                          frame Enabled {
                          }
                        }
                        n2208 = Multiply(x=w3911, y=w3909) -> (x*y=w3908:dbl)
                        n2209 = Subtract(x=w3908, y=272) -> (x-y=w3906:dbl)
                        "Amb Tp" <- w3906
                        n2210 = local write "Ref deg C"(w3906) -> ()
                        "deg C (volts)" <- w3909
                      }
                      frame True {
                      }
                    }
                  }
                }
              }
            }
          }
          frame #13 {
            # "save test data to file"
            n2211 = Get Date/Time In Seconds() -> (seconds since 1Jan1904=w3914:timestamp)
            "File Time Stamp" <- w3914
            n2212 = local read "on loops"() -> (w3933:dbl)
            n2213 = local read "jig cycle"() -> (w3930:dbl)
            n2214 = Format Date/Time String(time format string (%c)="%H:%M%:%S", seconds (now)=w3914) -> (date/time string=w3918:string)  [unwired: 1 in]
            n2215 = Add(x=w3933, y=2) -> (x+y=w3931:dbl)
            n2216 = Build Array(w3918) -> (w3917:string[])
